vi "Actor Core.vi"(8 "error in":errorcluster, 11 "VR-VNA_root in":refnum<class "VR-VNA_root.lvclass">) -> (0 "error out":errorcluster, 3 "Actor out":refnum<class "Actor.lvclass">)   [LabVIEW 2020, in "VR-VNA_root.lvlib" / "VR-VNA_root.lvclass"]
doc: "(<B>Filename</B>: Actor Framework.lvlib:Actor.lvclass:Actor Core.vi)\n\nReceives messages to the actor, reacts to them, and initiates any error handling that may shut the actor down.\n\nDescendant classes may override this VI to append parallel tasks for the actor to complete while it handles messages. Overrides use the Call Parent Class Method node."
uses:
  VR-VNA_root.lvclass
  <vilib>/ActorFramework/Actor/Actor.lvclass
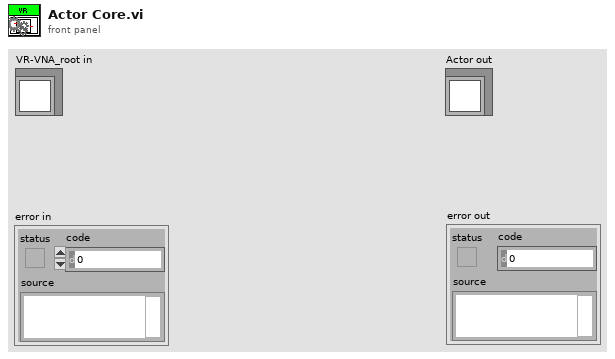
[diagram p1: front panel]
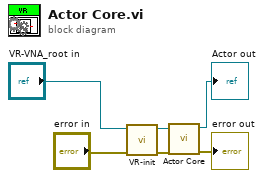
[diagram p0: block diagram]
diagram:
  n1 = call "VR-init.vi"("error in (no error)"="error in", "VR-VNA_root in"="VR-VNA_root in") -> ("error out"=w3:errorcluster, "VR-VNA_root out"=w4:refnum<class "VR-VNA_root.lvclass">)  [unwired: 8 in]
  n2 = call-parent "Actor Core.vi"("error in"=w3, "Actor in"=w4) -> ("error out"=→"error out":errorcluster, "Actor out"=→"Actor out":refnum<class "Actor.lvclass">)  [unwired: 8 in]
